vi "S2C_PCIe7841_Proc_ReadResourceName.vi"(8 "Error In":errorcluster) -> (0 "Error Out":errorcluster, 3 "ResourceName":string)   [LabVIEW 2015]
doc: "Reads the data contained within the Settings file and loads the data into VI specific global variables."
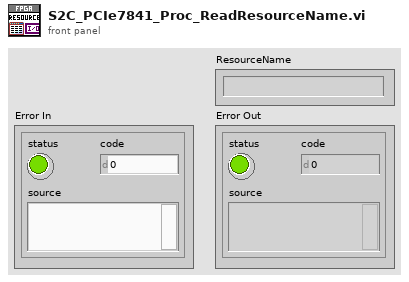
[diagram p1: front panel]
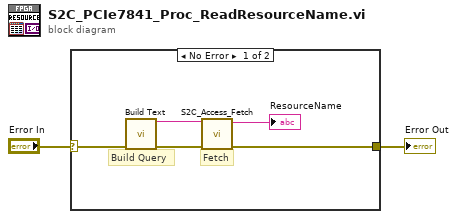
[diagram p0: block diagram]
diagram:
  n1 = case shown="No Error" "Error In" {
    selector: "Error In" -> [w5 w8]
    tunnel: [w4 w8] -> w1
    frame No Error {
      # "Fetch"
      # "Build Query"
      n2 = call "Build Text"("error in (no error)"=w5) -> ("Result"=w6:string, "error out"=w7:errorcluster)  [unwired: 13 in]
      n3 = call "S2C_Access_Fetch.vi"("Error In"=w7, "Query"=w6) -> ("Error Out"=w4:errorcluster, "Data"=→"ResourceName":string)  [unwired: 8 in]
    }
    frame Error {
    }
  }
  "Error Out" <- w1
